vi "ReadData_5782_with_cavity.vi"(10 "Buffer mode":T1, 11 "scope params":T2) -> (1 "Num elements":i32, 2 "data":dbl[][](array[numeric]) format="%.2f", 3 "scope params out":T2)   [LabVIEW 2013]
uses:
  controls/scope_params_5782.ctl
  Utilities/Ticker/Ticker.lvclass
  Communication/Driver/RemoteConnection/RemoteConnection.lvclass
  Scope/controls/ScopeMode.ctl
  Config/FPGAref_5782.ctl
  FPGA/DataMode.ctl
  controls/5782_trigger_type.ctl
  controls/Feedforward.ctl
  Scope/controls/Data_display_mode.ctl
  <vilib>/rvi/interface/common/niFpgaWaitOnOcc.vi
  <vilib>/Utility/error.llb/Error Cluster From Error Code.vi
  <vilib>/rvi/errors/niLvFpgaAdjustHostInterfaceError.vi
  <vilib>/rvi/interface/nirviMethod/nirviMethod.xnode
  <vilib>/FPGAPlugInAG/Dynamic/niLvFpga_ReadFifo_Dynamic.vi
  <vilib>/rvi/errors/niLvFpgaMergeErrorWithErrorCode.vi
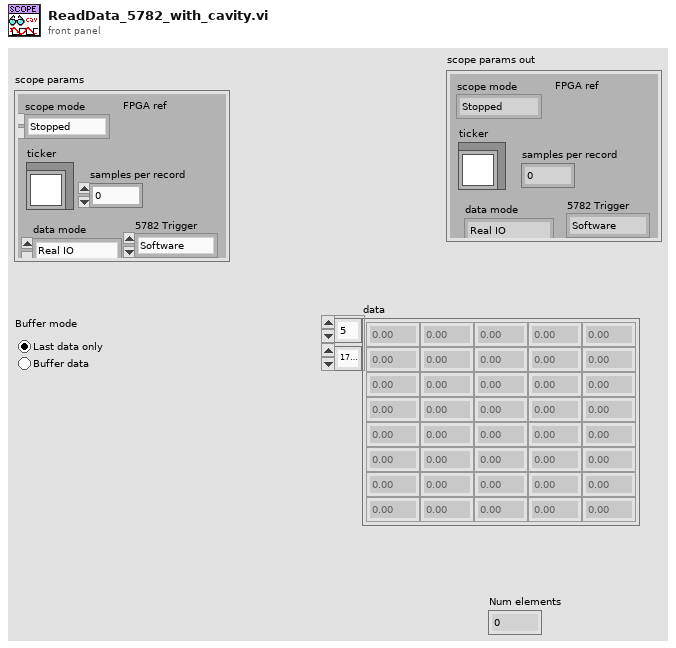
[diagram p1: front panel]
types:
  T1 = typedef "Data_display_mode.ctl" = enum32{"Last data only", "Buffer data"}
  T2 = typedef "scope_params_5782.ctl" = cluster{"scope mode":T3, "ticker":refnum<class "Ticker.lvclass">, "samples per record":i32, "FPGA ref":T4, "data mode":T5, "5782 Trigger":T6, "Chart length":i32, "RemoteConnection":refnum<class "RemoteConnection.lvclass">, "last phase":dbl[], "Feedforward":T7}
  T3 = typedef "ScopeMode.ctl" = enum16{"Stopped", "Single", "Running", "Continuous"}
  T4 = typedef "FPGAref_5782.ctl" = refnum<k20>
  T5 = typedef "DataMode.ctl" = enum16{"Real IO", "Simulated"}
  T6 = typedef "5782_trigger_type.ctl" = enum16{"Software", "Trigger input"}
  T7 = typedef "Feedforward.ctl" = cluster{"Beam I":dbl[], "Beam Q":dbl[], "Feedforward I":dbl[], "Feedforward Q":dbl[], "Setpoint I":dbl[], "Setpoint Q":dbl[]}
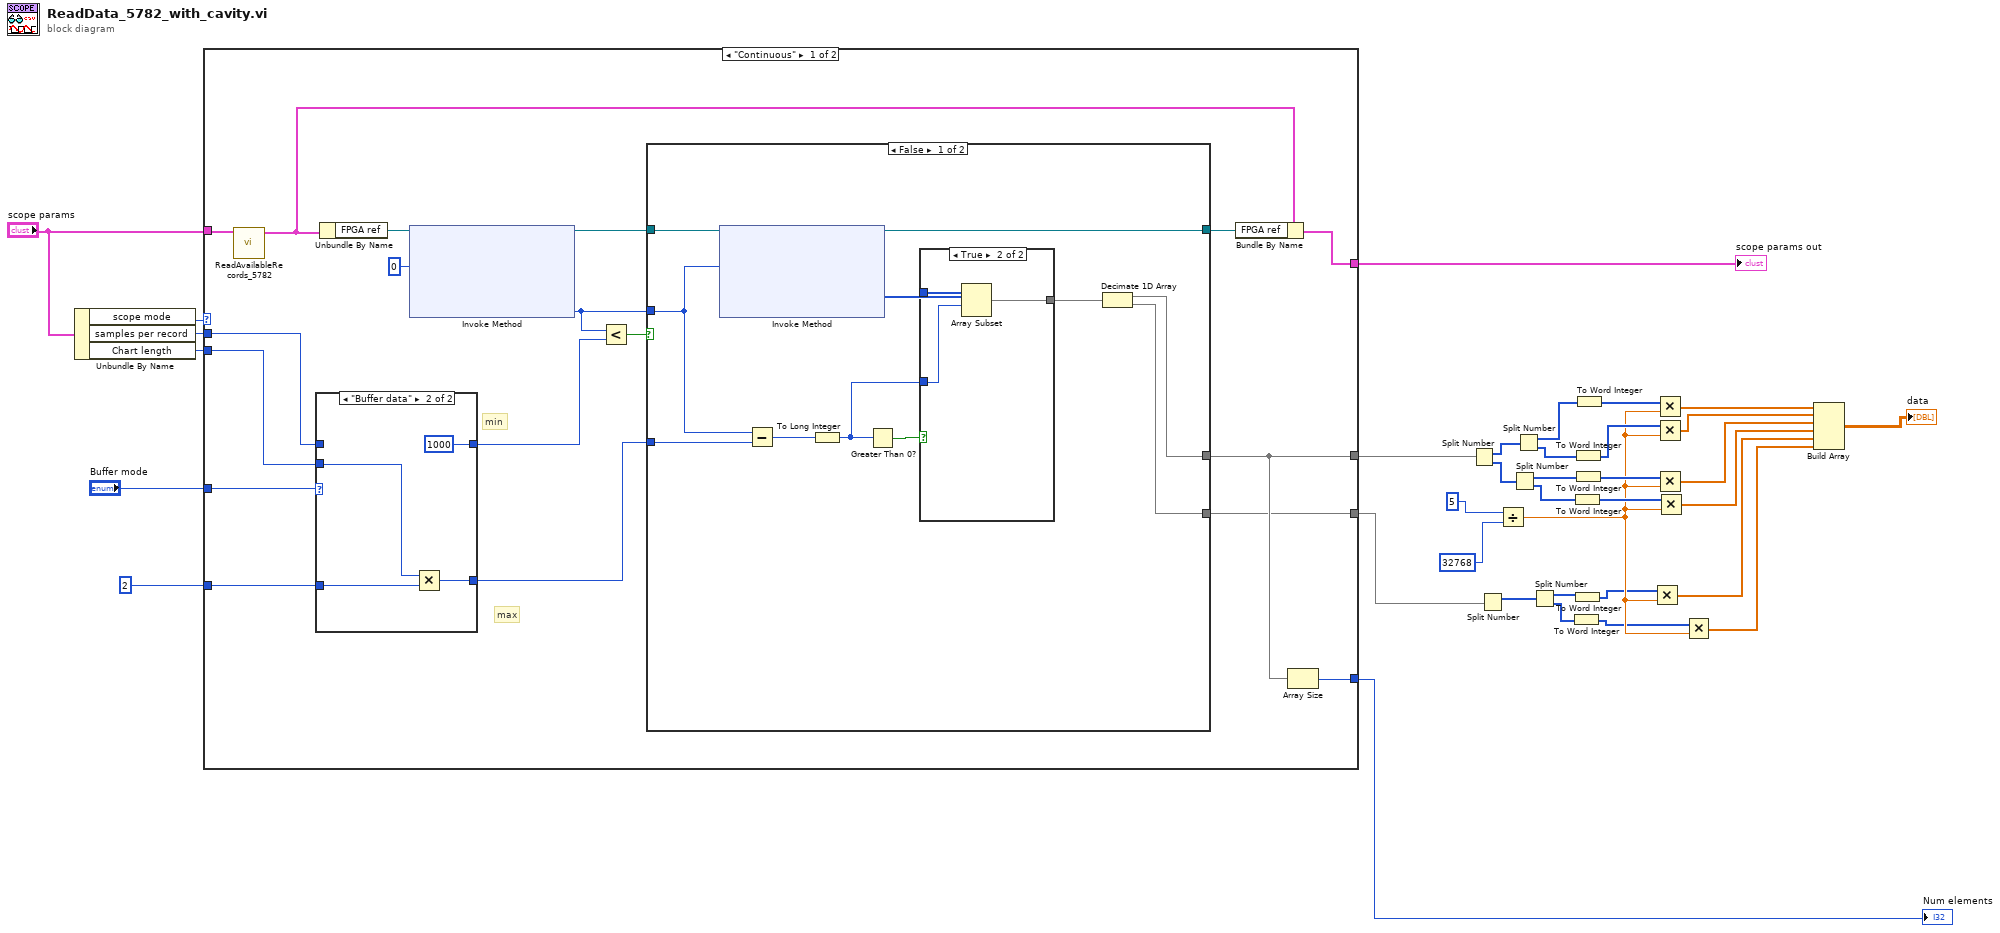
[diagram p0: block diagram]
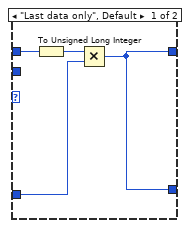
[diagram p4: hidden frame]
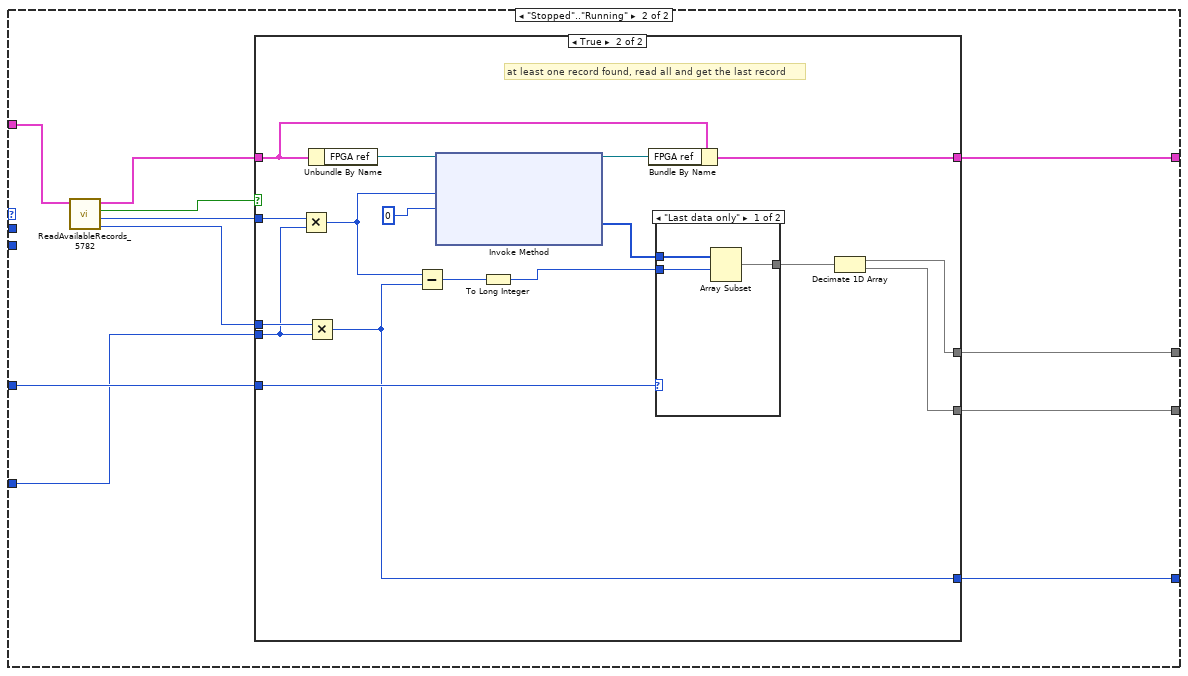
[diagram p5: hidden frame]
diagram:
  n1 = Unbundle By Name("scope params") -> ("scope mode"=w32:T3, "samples per record"=w29:i32, "Chart length"=w28:i32)
  n2 = case shown="\"Continuous\"" w32 {
    tunnel: [w42 w88] -> w35
    tunnel: [w44 w83] -> w34
    tunnel: [w43 w82] -> w30
    tunnel: "scope params" -> [w40 w81]
    tunnel: "Buffer mode" -> [w53 w80]
    tunnel: w29 -> [w41 _]
    tunnel: w28 -> [w38 _]
    tunnel: [w37 w79] -> w27
    tunnel: u32 2 ("y") -> [w36 w78]
    frame "Continuous" {
      # "min"
      # "max"
      n3 = call "ReadAvailableRecords_5782.vi"("scope params"=w40) -> ("scope params out"=w39:T2)  [unwired: 7 in, 3 out]
      n4 = case shown="\"Buffer data\"" w53 {
        tunnel: [w71 u32 1000] -> w50
        tunnel: [w71 w75] -> w46
        tunnel: w41 -> [w73 _]
        tunnel: w38 -> [_ w76]
        tunnel: w36 -> [w70 w74]
        frame "Last data only", Default {
          n5 = To Unsigned Long Integer(number=w73) -> (unsigned 32bit integer=w72:u32)
          n6 = Multiply(x=w72, y=w70) -> (x*y=w71:u32)
        }
        frame "Buffer data" {
          n7 = Multiply(x=w76, y=w74) -> (x*y=w75:u32)
        }
      }
      n8 = Unbundle By Name(w39) -> ("FPGA ref"=w52:T4)
      n9 = xnode "Invoke Method"("FPGA VI Reference In"=w52, "Number of Elements"=u32 0) -> ("FPGA VI Reference Out"=w48:T4, "Elements Remaining"=w47:u32)  [unwired: 2 in, 2 out]
      n10 = Less?(x=w47, y=w50) -> (x < y?=w49:bool)
      n11 = case shown="False" w49 {
        tunnel: w48 -> [w64 w69]
        tunnel: w47 -> [w62 _]
        tunnel: w46 -> [w61 _]
        tunnel: [w55 _] -> w43
        tunnel: [w58 w69] -> w45
        tunnel: [w54 _] -> w37
        frame False {
          n12 = xnode "Invoke Method"("FPGA VI Reference In"=w64, "Number of Elements"=w62) -> ("FPGA VI Reference Out"=w58:T4, "Data"=w57:u64[])  [unwired: 2 in, 2 out]
          n13 = Subtract(x=w62, y=w61) -> (x-y=w63:u32)
          n14 = To Long Integer(number=w63) -> (32bit integer=w59:i32)
          n15 = Greater Than 0?(x=w59) -> (x > 0?=w60:bool)
          n16 = case shown="True" w60 {
            tunnel: w57 -> [w65 w68]
            tunnel: w59 -> [_ w66]
            tunnel: [w65 w67] -> w56
            frame False {
            }
            frame True {
              n17 = Array Subset(array=w68, index=w66) -> (w67:u64[])  [unwired: 1 in]
            }
          }
          n18 = Decimate 1D Array(w56) -> (w55:u64[], w54:u64[])
        }
        frame True {
          # "too few elements"
        }
      }
      n19 = Bundle By Name(cluster=w39, "FPGA ref"=w45) -> (w44:T2)
      n20 = Array Size(array=w43) -> (size(s)=w42:i32)
    }
    frame "Stopped".."Running" {
      n21 = call "ReadAvailableRecords_5782.vi"("scope params"=w81) -> ("last record size"=w85:u32, "#elements"=w86:u32, "record available"=w87:bool, "scope params out"=w84:T2)  [unwired: 7 in]
      n22 = case shown="True" w87 {
        tunnel: [_ w95] -> w82
        tunnel: [_ w93] -> w88
        tunnel: w86 -> [_ w92]
        tunnel: w85 -> [_ w98]
        tunnel: w84 -> [w89 w104]
        tunnel: [w89 w100] -> w83
        tunnel: w80 -> [_ w99]
        tunnel: [_ w94] -> w79
        tunnel: w78 -> [_ w91]
        frame False {
        }
        frame True {
          # "at least one record found, read all and get the last record"
          n23 = Multiply(x=w92, y=w91) -> (x*y=w90:u32)
          n24 = Multiply(x=w98, y=w91) -> (x*y=w93:u32)
          n25 = Unbundle By Name(w104) -> ("FPGA ref"=w105:T4)
          n26 = Subtract(x=w90, y=w93) -> (x-y=w102:u32)
          n27 = xnode "Invoke Method"("FPGA VI Reference In"=w105, "Number of Elements"=w90, "Timeout (ms)"=0) -> ("FPGA VI Reference Out"=w103:T4, "Data"=w96:u64[])  [unwired: 1 in, 2 out]
          n28 = To Long Integer(number=w102) -> (32bit integer=w101:i32)
          n29 = Bundle By Name(cluster=w104, "FPGA ref"=w103) -> (w100:T2)
          n30 = case shown="\"Last data only\"" w99 {
            tunnel: w96 -> [w109 w110]
            tunnel: w101 -> [w107 _]
            tunnel: [w108 w110] -> w97
            frame "Last data only" {
              n31 = Array Subset(array=w109, index=w107) -> (w108:u64[])  [unwired: 1 in]
            }
            frame "Buffer data" {
            }
          }
          n32 = Decimate 1D Array(w97) -> (w95:u64[], w94:u64[])
        }
      }
    }
  }
  "scope params out" <- w34
  "Num elements" <- w35
  n33 = Split Number(x=w30) -> (hi(x)=w23:u32[], lo(x)=w19:u32[])
  n34 = Split Number(x=w27) -> (hi(x)=w7:u32[])  [unwired: 1 out]
  n35 = Divide(x=5, y=32768) -> (x/y=w6:dbl)
  n36 = Split Number(x=w19) -> (hi(x)=w21:u16[], lo(x)=w22:u16[])
  n37 = Split Number(x=w23) -> (hi(x)=w24:u16[], lo(x)=w20:u16[])
  n38 = Split Number(x=w7) -> (hi(x)=w4:u16[], lo(x)=w3:u16[])
  n39 = To Word Integer(number=w3) -> (16bit integer=w1:i16[])
  n40 = To Word Integer(number=w22) -> (16bit integer=w14:i16[])
  n41 = To Word Integer(number=w4) -> (16bit integer=w2:i16[])
  n42 = To Word Integer(number=w20) -> (16bit integer=w16:i16[])
  n43 = To Word Integer(number=w21) -> (16bit integer=w15:i16[])
  n44 = To Word Integer(number=w24) -> (16bit integer=w18:i16[])
  n45 = Multiply(x=w2, y=w6) -> (x*y=w9:dbl[])
  n46 = Multiply(x=w18, y=w6) -> (x*y=w17:dbl[])
  n47 = Multiply(x=w16, y=w6) -> (x*y=w13:dbl[])
  n48 = Multiply(x=w15, y=w6) -> (x*y=w12:dbl[])
  n49 = Multiply(x=w14, y=w6) -> (x*y=w11:dbl[])
  n50 = Multiply(x=w1, y=w6) -> (x*y=w10:dbl[])
  n51 = Build Array(w17, w13, w12, w11, w9, w10) -> (→"data":dbl[][])
